vi "Set Table Context.vi"(8 "error in (no error)":errorcluster, 9 "Context":T1, 10 "Table Names":string[](array[string]), 11 "Stack in":T1[](array[typedef])) -> (0 "error out":errorcluster, 3 "Stack out":T1[](array[typedef]))   [LabVIEW 2020, in "TOML.lvlib"]
uses:
  TOML.lvlib
  Context.ctl
  Table Context.ctl
  Key-Value Pair.ctl
  Value.ctl
  Value Type.ctl
  Table Array Context.ctl
  Add clue to error cluster.vi
  <vilib>/ErrorRing/Error Ring.xnode
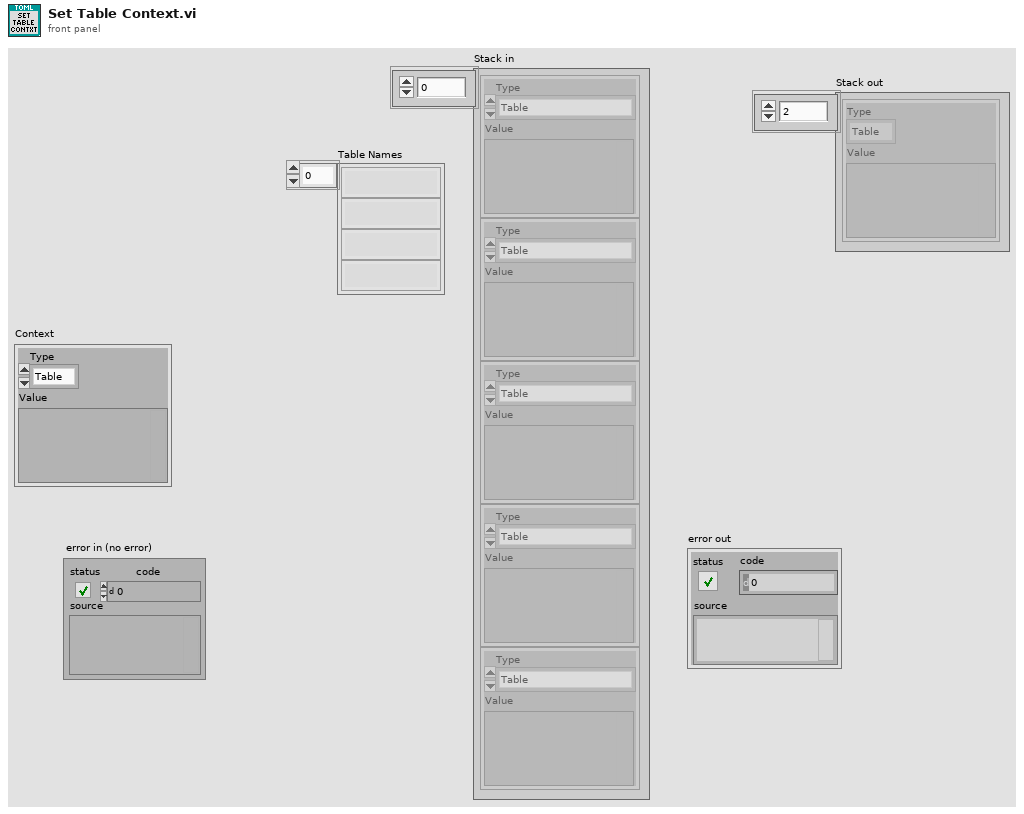
[diagram p1: front panel]
types:
  T1 = typedef "TOML.lvlib/Context.ctl" = cluster{"Type":enum16{"Table", "Array", "Inline Table", "Table Array"}, "Value":variant}
  T2 = enum16{"Table", "Array", "Inline Table", "Table Array"}
  T3 = typedef "TOML.lvlib/Table Context.ctl" = cluster{"Table":T4[], "Key":string, "Defined Keys":string[]}
  T4 = typedef "TOML.lvlib/Key-Value Pair.ctl" = cluster{"Key":string, "Value":T5}
  T5 = typedef "TOML.lvlib/Value.ctl" = cluster{"Type":T6, "Value":variant}
  T6 = typedef "TOML.lvlib/Value Type.ctl" = enum16{"Table", "Array", "String", "Integer", "Float", "Boolean", "Offset Date-Time", "Local Date-Time", "Local Date", "Local Time", "Path"}
  T7 = typedef "TOML.lvlib/Table Array Context.ctl" = cluster{"Table Array":cluster{"Table":T4[]}[], "Index":i32, "Key":string}
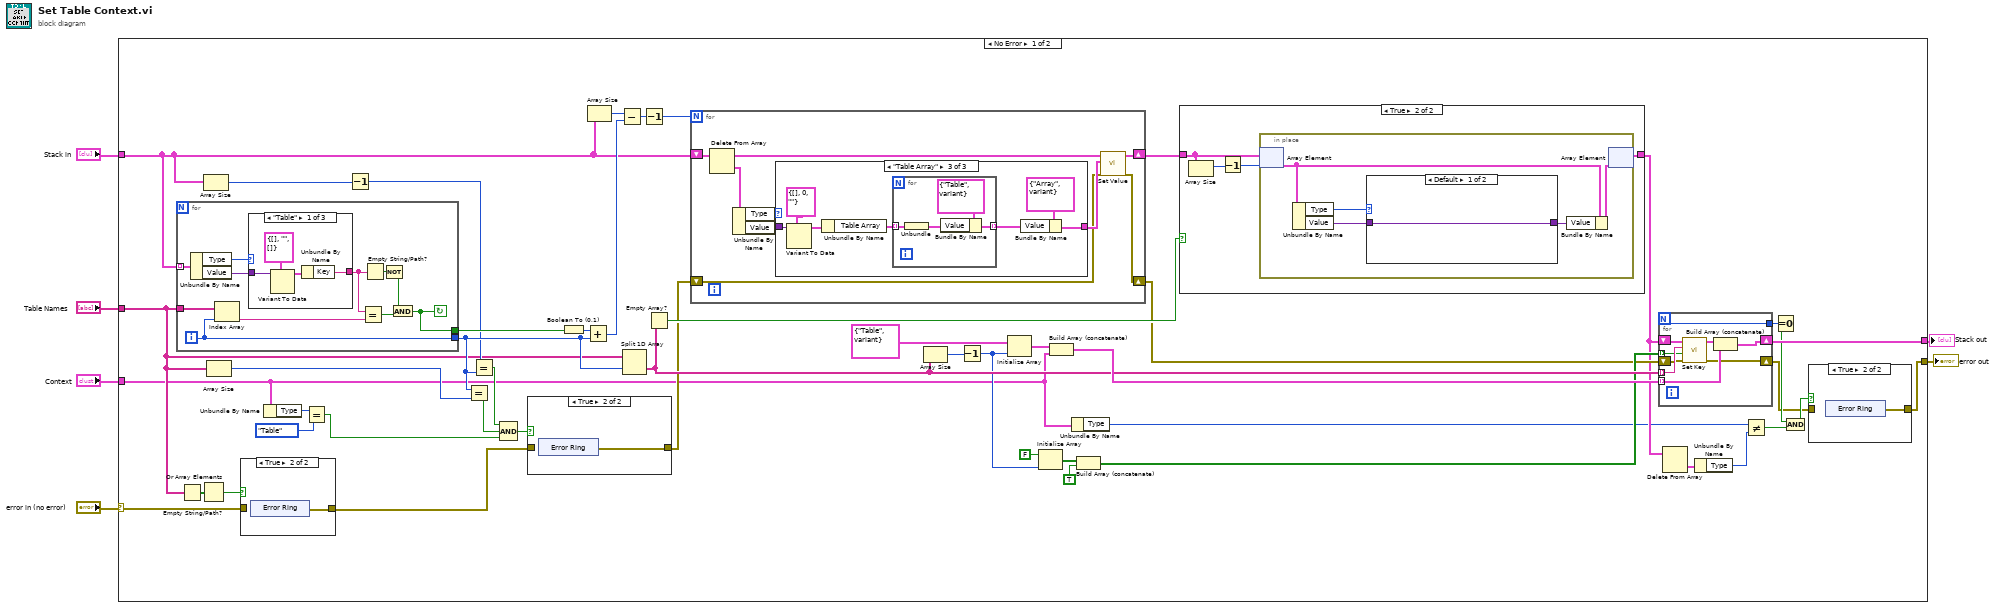
[diagram p0: block diagram]
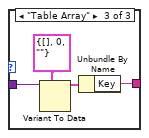
[diagram p5: hidden frame]
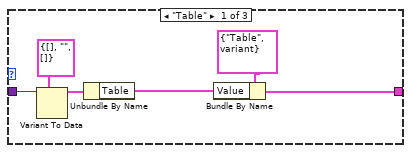
[diagram p7: hidden frame]
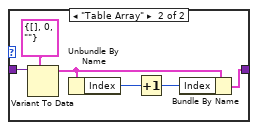
[diagram p10: hidden frame]
diagram:
  n1 = case shown="No Error" "error in (no error)" {
    selector: "error in (no error)" -> [w19 w135]
    tunnel: [w49 w136] -> w6
    tunnel: "Context" -> [w17 _]
    tunnel: [w9 w135] -> w4
    tunnel: "Table Names" -> [w22 _]
    tunnel: "Stack in" -> [w34 w136]
    frame No Error {
      n2 = for {
        tunnel: w34 -> [w70] mode=indexing
        tunnel: w22 -> [w71]
        tunnel: [w63] -> w31
        tunnel: [w62] -> w54
        i -> [w63]
        stop <- w62 continue-if-true
        n3 = Unbundle By Name(w70) -> ("Type"=w69:T2, "Value"=w68:variant)
        n4 = Index Array(array=w71, index=w63) -> (element=w67:string)
        n5 = case shown="\"Table\"" w69 {
          tunnel: w68 -> [w75 _ w79]
          tunnel: [w72 _ w76] -> w66
          frame "Table" {
            n6 = Variant To Data(type=T3 {"Table"=[], "Key"="", "Defined Keys"=[]} ("Table Context"), Variant=w75) -> (data=w73:T3)  [unwired: 1 in, 1 out]
            n7 = Unbundle By Name(w73) -> ("Key"=w72:string)
          }
          frame Default {
          }
          frame "Table Array" {
            n8 = Variant To Data(type=T7 {"Table Array"=[], "Index"=0, "Key"=""} ("Table Array Context"), Variant=w79) -> (data=w77:T7)  [unwired: 1 in, 1 out]
            n9 = Unbundle By Name(w77) -> ("Key"=w76:string)
          }
        }
        n10 = Equal?(x=w66, y=w67) -> (x = y?=w65:bool)
        n11 = Empty String/Path?(string/path=w66) -> (empty?=w64:bool)
        n12 = Not(x=w64) -> (.not. x?=w61:bool)
        n13 = And(x=w61, y=w65) -> (x .and. y?=w62:bool)
      }
      n14 = Empty String/Path?(string/path=w22) -> (empty?=w21:bool[])
      n15 = Or Array Elements(Boolean array=w21) -> (logical OR=w7:bool)
      n16 = Array Size(array=w34) -> (size(s)=w32:i32)
      n17 = Array Size(array=w22) -> (size(s)=w33:i32)
      n18 = case shown="True" w7 {
        tunnel: [w55 w56] -> w20
        tunnel: w19 -> [w55 _]
        frame False {
        }
        frame True {
          n19 = xnode "Error Ring"() -> ("error out"=w56:errorcluster)
        }
      }
      n20 = Unbundle By Name(w17) -> ("Type"=w25:T2)
      n21 = Equal?(x=w25, y=T2."Table") -> (x = y?=w23:bool)
      n22 = Decrement(x=w32) -> (x-1=w26:i32)
      n23 = Equal?(x=w31, y=w33) -> (x = y?=w29:bool)
      n24 = Equal?(x=w26, y=w31) -> (x = y?=w28:bool)
      n25 = Compound Arithmetic op=AND(w28, w29, w23) -> (w30:bool)
      n26 = case shown="True" w30 {
        tunnel: w20 -> [w58 _]
        tunnel: [w58 w59] -> w27
        frame False {
        }
        frame True {
          n27 = xnode "Error Ring"() -> ("error out"=w59:errorcluster)
        }
      }
      n28 = Boolean To (0,1)(Boolean=w54) -> (0, 1=w53:i16)
      n29 = Add(x=w53, y=w31) -> (x+y=w50:i32)
      n30 = Array Size(array=w34) -> (size(s)=w52:i32)
      n31 = Subtract(x=w52, y=w50) -> (x-y=w51:i32)
      n32 = Split 1D Array(array=w22, index=w31) -> (second subarray=w43:string[])  [unwired: 1 out]
      n33 = Decrement(x=w51) -> (x-1=w48:i32)
      n34 = Empty Array?(array=w43) -> (empty?=w41:bool)
      n35 = for {
        N: w48 -> [_]
        shift-right: [w86] -> w42
        shift-left: w34 -> [w91]
        shift-right: [w83] -> w35
        shift-left: w27 -> [w84]
        n36 = Delete From Array(array=w91) -> (deleted portion=w88:T1, array with subset deleted=w87:T1[])  [unwired: 2 in]
        n37 = Unbundle By Name(w88) -> ("Type"=w89:T2, "Value"=w90:variant)
        n38 = case shown="\"Table Array\"" w89 {
          tunnel: w90 -> [w97 _ w104]
          tunnel: [w92 _ w98] -> w85
          frame "Table" {
            n39 = Variant To Data(type=T3 {"Table"=[], "Key"="", "Defined Keys"=[]} ("Table Context"), Variant=w97) -> (data=w95:T3)  [unwired: 1 in, 1 out]
            n40 = Unbundle By Name(w95) -> ("Table"=w93:T4[])
            n41 = Bundle By Name(cluster=T5 {"Type"=enum."Table", "Value"=variant} ("Value"), "Value"=w93) -> (w92:T5)
          }
          frame Default {
          }
          frame "Table Array" {
            n42 = Variant To Data(type=T7 {"Table Array"=[], "Index"=0, "Key"=""} ("Table Array Context"), Variant=w104) -> (data=w102:T7)  [unwired: 1 in, 1 out]
            n43 = Unbundle By Name(w102) -> ("Table Array"=w101:cluster{"Table":T4[]}[])
            n44 = for {
              tunnel: w101 -> [w108] mode=indexing
              tunnel: [w105] -> w99 mode=indexing
              n45 = Unbundle(w108) -> ("Table"=w106:T4[])
              n46 = Bundle By Name(cluster=T5 {"Type"=enum."Table", "Value"=variant} ("Value"), "Value"=w106) -> (w105:T5)
            }
            n47 = Bundle By Name(cluster=T5 {"Type"=enum."Array", "Value"=variant} ("Value"), "Value"=w99) -> (w98:T5)
          }
        }
        n48 = call "Set Value.vi"("error in (no error)"=w84, "Value"=w85, "Context in"=w87) -> ("error out"=w83:errorcluster, "Context out"=w86:T1[])  [unwired: 5 in, 2 out]
      }
      n49 = Array Size(array=w43) -> (size(s)=w47:i32)
      n50 = Decrement(x=w47) -> (x-1=w40:i32)
      n51 = Initialize Array(T1 {"Type"=enum."Table", "Value"=variant} ("Context"), w40) -> (w45:T1[])
      n52 = Initialize Array(FALSE, w40) -> (w38:bool[])
      n53 = Build Array (concatenate)(w45, w17) -> (w44:T1[])
      n54 = Unbundle By Name(w17) -> ("Type"=w13:T2)
      n55 = Build Array (concatenate)(w38, TRUE) -> (w36:bool[])
      n56 = case shown="True" w41 {
        tunnel: w42 -> [w109 w113]
        tunnel: [w109 w112] -> w16
        frame False {
        }
        frame True {
          n57 = Array Size(array=w113) -> (size(s)=w111:i32)
          n58 = Decrement(x=w111) -> (x-1=w110:i32)
          n59 = in-place {
            n60 = in-place-array #1(w113, w110) -> (w116:T1)
            n61 = Unbundle By Name(w116) -> ("Type"=w118:T2, "Value"=w117:variant)
            n62 = case shown="Default" w118 {
              tunnel: w117 -> [w119 w125]
              tunnel: [w119 w120] -> w115
              frame Default {
              }
              frame "Table Array" {
                n63 = Variant To Data(type=T7 {"Table Array"=[], "Index"=0, "Key"=""} ("Table Array Context"), Variant=w125) -> (data=w123:T7)  [unwired: 1 in, 1 out]
                n64 = Unbundle By Name(w123) -> ("Index"=w121:i32)
                n65 = Increment(x=w121) -> (x+1=w122:i32)
                n66 = Bundle By Name(cluster=w123, "Index"=w122) -> (w120:T7)
              }
            }
            n67 = Bundle By Name(cluster=w116, "Value"=w115) -> (w114:T1)
            n68 = in-place-array #1(w114) -> (w112:T1[])  [unwired: 1 out]
          }
        }
      }
      n69 = for {
        N -> [w126]
        shift-right: [w132] -> w49
        shift-left: w16 -> [w134]
        tunnel: w43 -> [w133] mode=indexing
        tunnel: w44 -> [w131] mode=indexing
        tunnel: w36 -> [w129] mode=indexing
        shift-right: [w127] -> w8
        shift-left: w35 -> [w128]
        tunnel: [w126] -> w18
        n70 = call "Set Key.vi"("error in (no error)"=w128, "Define"=w129, "Key"=w133, "Stack in"=w134) -> ("error out"=w127:errorcluster, "Stack out"=w130:T1[])  [unwired: 6 in]
        n71 = Build Array (concatenate)(w130, w131) -> (w132:T1[])
      }
      n72 = Delete From Array(array=w16) -> (deleted portion=w15:T1)  [unwired: 2 in, 1 out]
      n73 = Unbundle By Name(w15) -> ("Type"=w14:T2)
      n74 = Not Equal?(x=w13, y=w14) -> (x != y?=w12:bool)
      n75 = Equal To 0?(x=w18) -> (x = 0?=w11:bool)
      n76 = And(x=w11, y=w12) -> (x .and. y?=w10:bool)
      n77 = case shown="True" w10 {
        tunnel: [w80 w81] -> w9
        tunnel: w8 -> [w80 _]
        frame False {
        }
        frame True {
          n78 = xnode "Error Ring"() -> ("error out"=w81:errorcluster)
        }
      }
    }
    frame Error {
    }
  }
  "Stack out" <- w6
  "error out" <- w4
